vi "CRYCheck Empty Data.vi"(10 "Step No":i32=-1, 11 "Type":enum16{"Curves", "Values", "Results", "WFM"}(ring)) -> (3 "NoEmpty?":bool)   [LabVIEW 2013]
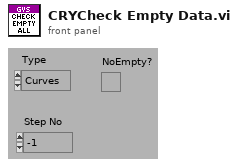
[diagram p1: front panel]
types:
  T1 = typedef "CRYData Cluster.ctl" = cluster{"Name":string, "Curve":cluster{"x":dbl, "y":dbl, "z":dbl}[], "X data":u16, "Y data":u16, "Z data":u16, "X axis":u16, "Y axis":u16, "Z axis":u16, "X unit":string, "Y unit":string, "Z unit":string, "X dB ref":dbl, "Y dB ref":dbl, "Z dB ref":dbl, "single val":bool, "protected":bool, "display X":bool, "display Y":bool, "display Z":bool, "Test Info":string, "Step No.":i32, "Plot Settings":cluster{"Color":u32, "Interpolation":u8, "Point Style":u8, "Line Style":u8, "Point Color":u32, "Line Width":u8, "Bar Plot Style":u8, "Fill To":i16}, "AutoProtect":bool}
  T2 = typedef "CRYWaveform Cluster.ctl" = cluster{"Waveform":cluster{"X0":dbl, "dX":dbl, "Y":sgl[]}, "X data":u16, "Y data":u16, "Y axis":u16, "X unit":string, "Y unit":string, "Y dB ref":dbl, "display Y":bool, "display X":bool, "Overload?":bool, "Test Info":string, "Step No.":i32, "Name":string, "protected":bool, "Sqc history":string[], "Signal Channel ID":i32, "Plot Settings":cluster{"Color":u32, "Interpolation":u8, "Point Style":u8, "Line Style":u8, "Point Color":u32, "Line Width":u8, "Bar Plot Style":u8, "Fill To":i16}, "AutoProtect":bool}
  T3 = typedef "CRYResult Cluster.ctl" = cluster{"Name":string, "Margin":dbl, "unit":string, "Verdict":bool, "Limit":string, "Max/Min":string, "protected":bool, "Step No.":i32, "Test Info":string, "AutoProtect":bool}
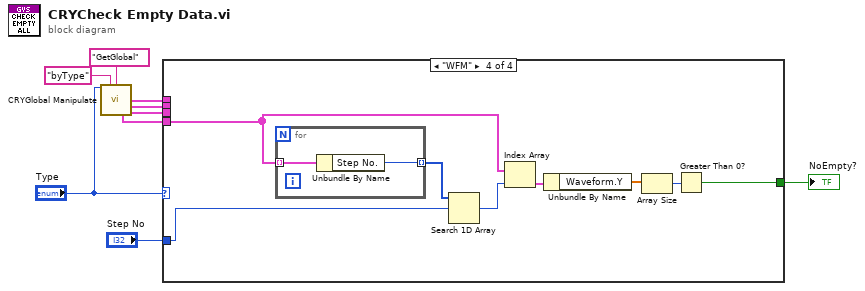
[diagram p0: block diagram]
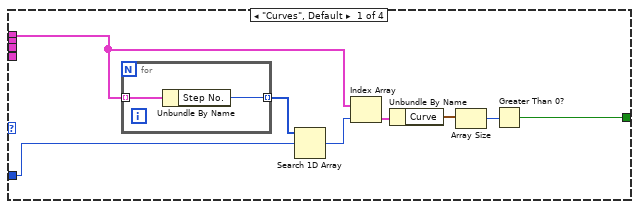
[diagram p2: hidden frame]
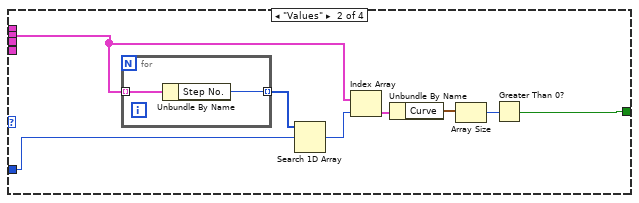
[diagram p3: hidden frame]
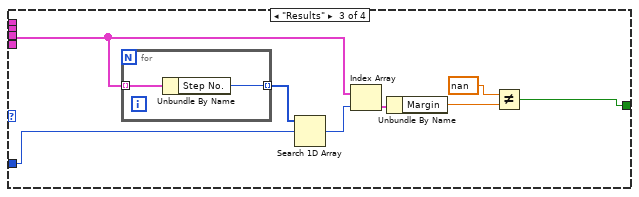
[diagram p4: hidden frame]
diagram:
  n1 = call "CRYGlobal Manipulate.vi"("Type"="Type", "sOption"="byType", "sAction"="GetGlobal") -> ("Curves Out"=w6:T1[], "Values Out"=w5:T1[], "WFM Out"=w3:T2[], "Results Out"=w4:T3[])  [unwired: 6 in, 3 out]
  n2 = case shown="\"WFM\"" "Type" {
    tunnel: "Step No" -> [w15 w25 w35 w45]
    tunnel: [w11 w21 w31 w41] -> w8
    tunnel: w6 -> [w10 _ _ _]
    tunnel: w5 -> [_ w20 _ _]
    tunnel: w4 -> [_ _ w30 _]
    tunnel: w3 -> [_ _ _ w40]
    frame "Curves", Default {
      n3 = for {
        tunnel: w10 -> [w19] mode=indexing
        tunnel: [w18] -> w17 mode=indexing
        n4 = Unbundle By Name(w19) -> ("Step No."=w18:i32)
      }
      n5 = Search 1D Array(1D array=w17, element=w15) -> (index of element=w16:i32)  [unwired: 1 in]
      n6 = Index Array(array=w10, index=w16) -> (element=w14:T1)
      n7 = Unbundle By Name(w14) -> ("Curve"=w13:cluster{"x":dbl, "y":dbl, "z":dbl}[])
      n8 = Array Size(array=w13) -> (size(s)=w12:i32)
      n9 = Greater Than 0?(x=w12) -> (x > 0?=w11:bool)
    }
    frame "Values" {
      n10 = for {
        tunnel: w20 -> [w29] mode=indexing
        tunnel: [w28] -> w27 mode=indexing
        n11 = Unbundle By Name(w29) -> ("Step No."=w28:i32)
      }
      n12 = Search 1D Array(1D array=w27, element=w25) -> (index of element=w26:i32)  [unwired: 1 in]
      n13 = Index Array(array=w20, index=w26) -> (element=w24:T1)
      n14 = Unbundle By Name(w24) -> ("Curve"=w23:cluster{"x":dbl, "y":dbl, "z":dbl}[])
      n15 = Array Size(array=w23) -> (size(s)=w22:i32)
      n16 = Greater Than 0?(x=w22) -> (x > 0?=w21:bool)
    }
    frame "Results" {
      n17 = for {
        tunnel: w30 -> [w39] mode=indexing
        tunnel: [w38] -> w37 mode=indexing
        n18 = Unbundle By Name(w39) -> ("Step No."=w38:i32)
      }
      n19 = Search 1D Array(1D array=w37, element=w35) -> (index of element=w36:i32)  [unwired: 1 in]
      n20 = Index Array(array=w30, index=w36) -> (element=w34:T3)
      n21 = Unbundle By Name(w34) -> ("Margin"=w33:dbl)
      n22 = Not Equal?(x=nan ("Margin"), y=w33) -> (x != y?=w31:bool)
    }
    frame "WFM" {
      n23 = for {
        tunnel: w40 -> [w49] mode=indexing
        tunnel: [w48] -> w47 mode=indexing
        n24 = Unbundle By Name(w49) -> ("Step No."=w48:i32)
      }
      n25 = Search 1D Array(1D array=w47, element=w45) -> (index of element=w46:i32)  [unwired: 1 in]
      n26 = Index Array(array=w40, index=w46) -> (element=w44:T2)
      n27 = Unbundle By Name(w44) -> ("Waveform.Y"=w43:sgl[])
      n28 = Array Size(array=w43) -> (size(s)=w42:i32)
      n29 = Greater Than 0?(x=w42) -> (x > 0?=w41:bool)
    }
  }
  "NoEmpty?" <- w8
